vi "error.vi"(7 "stop":bool, 11 "Qube":refnum<class "Qube.lvclass">) -> (0 "abort?":bool, 3 "Qube":refnum<class "Qube.lvclass">)   [LabVIEW 2017, in "Qube.lvclass"]
uses:
  Qube.lvclass
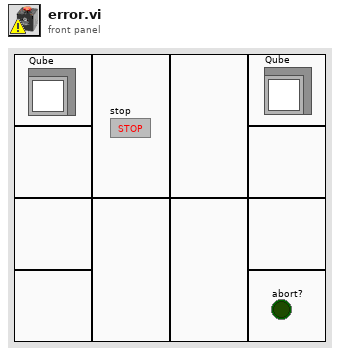
[diagram p1: front panel]
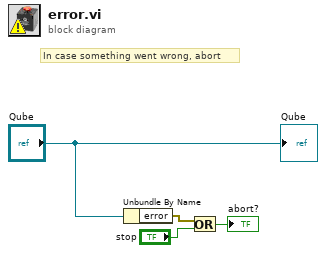
[diagram p0: block diagram]
diagram:
  # "In case something went wrong, abort"
  n1 = Unbundle By Name("Qube") -> ("error"=w4:errorcluster)
  n2 = Or(x=w4, y="stop") -> (x .or. y?=→"abort?":bool)
  "Qube" <- "Qube"
